vi "ControlFunction.vi"(8 "error in (no error)":errorcluster, 11 "CubeLift in":refnum<class "CubeLift.lvclass">) -> (0 "error out":errorcluster, 3 "CubeLift out":refnum<class "CubeLift.lvclass">)   [LabVIEW 2017, in "CubeLift.lvclass"]
uses:
  CubeLift.lvclass
  SubsystemData/CubeLiftData/CubeLiftData.lvclass
  R:/Documents/github/FRC4080/2018-robot-main/SubsystemData/SubsystemData.lvclass
  CubeLift.lvclass/CubeLift.ctl
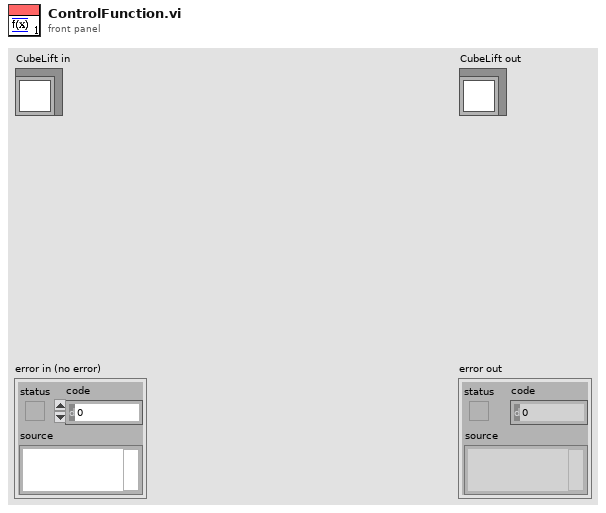
[diagram p1: front panel]
types:
  T1 = typedef "CubeLiftData.lvclass/CubeLiftCommand.ctl" = cluster{"Bucket":cluster{"Deposit":bool}, "Slide":cluster{"Slide command":enum16{"Up", "Down", "Stationary"}}}
  T2 = typedef "CubeLiftData.lvclass/CubeLiftOutput.ctl" = cluster{"LiftOutputSetting":dbl, "DepositCube?":bool, "LiftControlMode":T3}
  T3 = typedef "CTRE_Phoenix_MotorControl_ControlMode.ctl" = u16
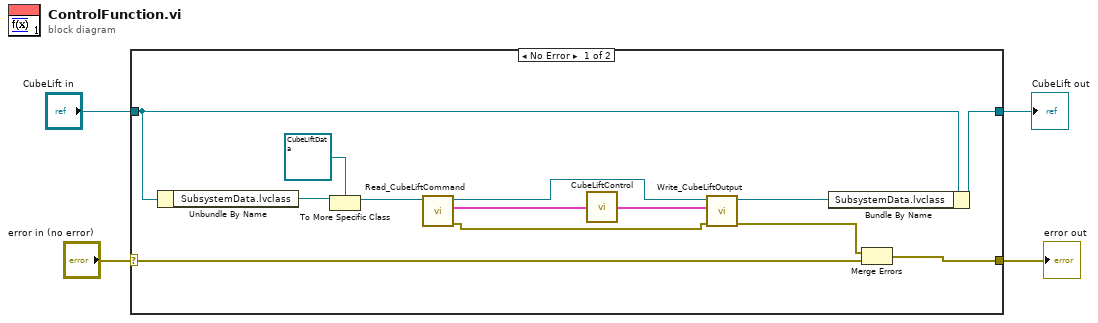
[diagram p0: block diagram]
diagram:
  n1 = case shown="No Error" "error in (no error)" {
    selector: "error in (no error)" -> [w17 w19]
    tunnel: [w6 w19] -> w3
    tunnel: [w15 w18] -> w1
    tunnel: "CubeLift in" -> [w16 w18]
    frame No Error {
      n2 = Unbundle By Name(w16) -> ("SubsystemData.lvclass"=w14:refnum<class "SubsystemData.lvclass">)
      n3 = To More Specific Class(target class=refnum<class "CubeLiftData.lvclass"> refnum ("CubeLiftData.lvclass"), reference=w14) -> (specific class reference=w12:refnum<class "CubeLiftData.lvclass">)  [unwired: 1 in, 1 out]
      n4 = call-dynamic "Read_CubeLiftCommand.vi"("CubeLiftData in"=w12) -> ("error out"=w9:errorcluster, "Cube Lift Command"=w7:T1, "CubeLiftData out"=w10:refnum<class "CubeLiftData.lvclass">)  [unwired: 8 in]
      n5 = call "CubeLiftControl.vi"("Cube Lift Command"=w7) -> ("CubeLiftOutput"=w11:T2)  [unwired: 6 in]
      n6 = call-dynamic "Write_CubeLiftOutput.vi"("error in (no error)"=w9, "CubeLiftOutput"=w11, "CubeLiftData in"=w10) -> ("error out"=w5:errorcluster, "CubeLiftData out"=w8:refnum<class "CubeLiftData.lvclass">)  [unwired: 7 in]
      n7 = Bundle By Name(cluster=w16, "SubsystemData.lvclass"=w8) -> (w15:refnum<class "CubeLift.lvclass">)
      n8 = Merge Errors(w5, w17) -> (w6:errorcluster)
    }
    frame Error {
    }
  }
  "error out" <- w3
  "CubeLift out" <- w1
